vi "Vent_solenoid_EC_subVI_BM.vi"(8 "BoardNum":u32=42, 10 "BitNum":u32=2, 11 "Vent?":bool) -> (3 "Vented":bool)   [LabVIEW 2021]
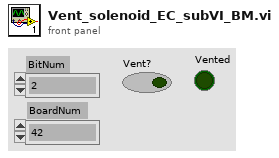
[diagram p1: front panel]
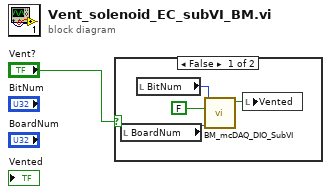
[diagram p0: block diagram]
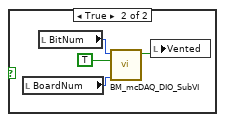
[diagram p2: hidden frame]
diagram:
  n1 = case shown="False" "Vent?" {
    frame False {
      n2 = local read "BoardNum"() -> (w3:u32)
      n3 = local read "BitNum"() -> (w2:u32)
      n4 = call "BM_mcDAQ_DIO_SubVI.vi"("BoardNum"=w3, "BitValue"=FALSE, "BitNum"=w2) -> ("Control out"=w4:bool)  [unwired: 8 in]
      n5 = local write "Vented"(w4) -> ()
    }
    frame True {
      n6 = local read "BoardNum"() -> (w6:u32)
      n7 = local read "BitNum"() -> (w7:u32)
      n8 = call "BM_mcDAQ_DIO_SubVI.vi"("BoardNum"=w6, "BitValue"=TRUE, "BitNum"=w7) -> ("Control out"=w8:bool)  [unwired: 8 in]
      n9 = local write "Vented"(w8) -> ()
    }
  }
